vi "Seconds Wait.vi"(2 "Point #":i32, 3 "Parameters":dbl[](array[numeric]) format="%.3e") -> (0 "Stop":bool, 1 "Time Stamp (Sec)":dbl[](array[numeric]) format="%.2f")   [LabVIEW 2020]
doc: "Returns time in seconds since point number zero. After the time stamp is calculated, the program waits for the requisite # of seconds specified by the first parameter.\nScott Hannahs, NHMFL/FSU, Feb 1996"
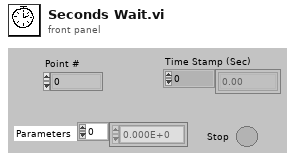
[diagram p1: front panel]
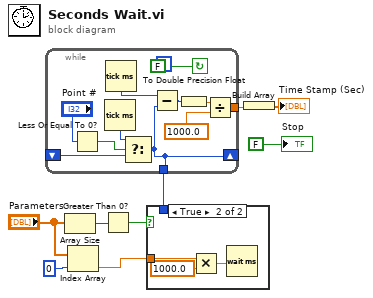
[diagram p0: block diagram]
diagram:
  n1 = while {
    tunnel: [w11] -> w4
    tunnel: [w15] -> w9
    shift-left: _ -> [w18]
    shift-right: [w11] -> _
    stop <- FALSE continue-if-true
    n2 = Less Or Equal To 0?(x="Point #") -> (x <= 0?=w19:bool)
    n3 = Tick Count (ms)() -> (millisecond timer value=w17:u32)
    n4 = Tick Count (ms)() -> (millisecond timer value=w16:u32)
    n5 = Select(t=w17, s=w19, f=w18) -> (s? t:f=w11:u32)
    n6 = Subtract(x=w16, y=w11) -> (x-y=w13:u32)
    n7 = To Double Precision Float(number=w13) -> (double precision float=w12:dbl)
    n8 = Divide(x=w12, y=1000.0) -> (x/y=w15:dbl)
  }
  n9 = Array Size(array="Parameters") -> (size(s)=w6:i32)
  n10 = Index Array(array="Parameters", index=0) -> (element=w1:dbl)
  n11 = Greater Than 0?(x=w6) -> (x > 0?=w5:bool)
  n12 = case shown="True" w5 {
    tunnel: w4 -> [_ _]
    tunnel: w1 -> [_ w22]
    frame False {
    }
    frame True {
      n13 = Multiply(x=w22, y=1000.0) -> (x*y=w21:dbl)
      n14 = Wait (ms)(milliseconds to wait=w21) -> ()  [unwired: 1 out]
    }
  }
  n15 = Build Array(w9) -> (→"Time Stamp (Sec)":dbl[])
  "Stop" <- FALSE
